vi "happiness.vi"(1 "T_room":dbl) -> (0 "Happiness [%]":dbl(slide) scale=0.0..100.0)   [LabVIEW 2014]
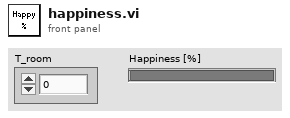
[diagram p1: front panel]
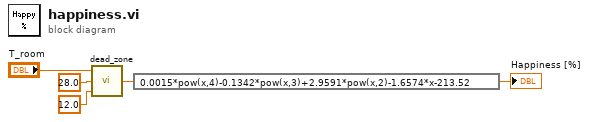
[diagram p0: block diagram]
diagram:
  n1 = call "dead_zone.vi"("min"=12.0, "max"=28.0, "number in"="T_room") -> ("number out"=w5:dbl)
  n2 = expression code="0.0015*pow(x,4)-0.1342*pow(x,3)+2.9591*pow(x,2)-1.6574*x-213.52"(w5) -> (→"Happiness [%]":dbl)
